vi "Test LakeShore 340.vi"(8 "error in (no error)":errorcluster, 11 "VISA Resource Name":refnum<visa-resource-name>) -> (0 "error out":errorcluster, 2 "Heater%":dbl, 3 "VISA Resource Name Out":refnum<visa-resource-name>)   [LabVIEW 2024]
panel:
  out "read buffer":string
  in  "byte count":u32
  out "Raw 2":dbl
  out "Temperature 2":dbl
  in  "Set point":dbl format="%.2f"
  in  "Output #":i32=1
  out "Raw":dbl
  out "Temperature":dbl
  in  "Input (A or B)":string="A"
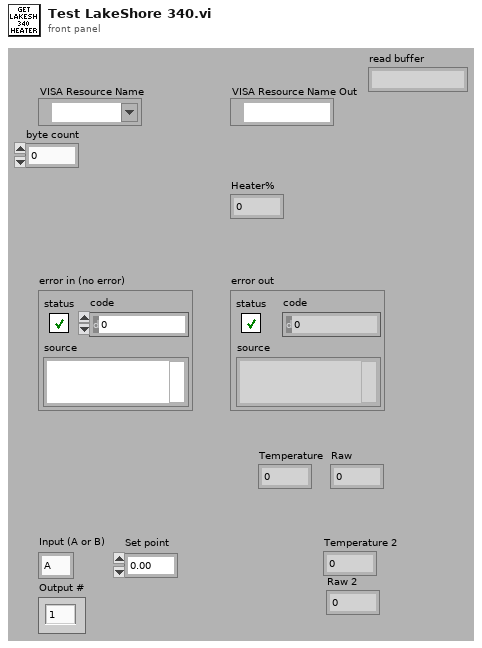
[diagram p1: front panel]
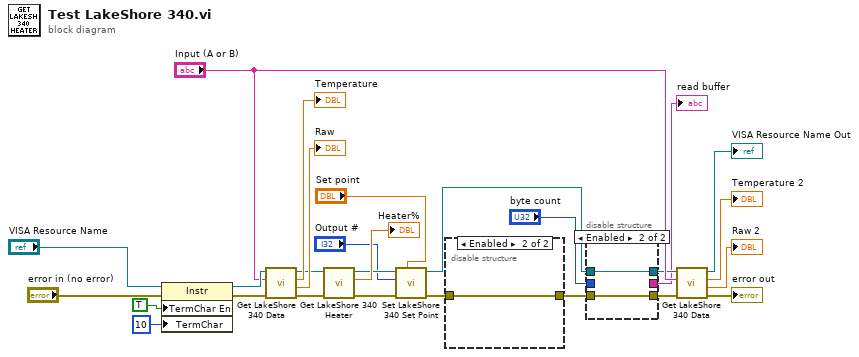
[diagram p0: block diagram]
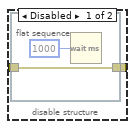
[diagram p2: hidden frame]
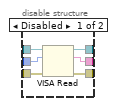
[diagram p3: hidden frame]
diagram:
  n1 = property class="Instr"(reference="VISA Resource Name", error in="error in (no error)", "TermChar En"=TRUE ("Message Based Settings:Termination Character Enable"), "TermChar"=u8 10 ("Message Based Settings:Termination Character")) -> (reference out=w23:refnum<visa-resource-name>, error out=w22:errorcluster)
  n2 = call "Get LakeShore 340 Data.vi"("error in (no error)"=w22, "Input (A or B)"="Input (A or B)", "VISA Resource Name"=w23) -> ("error out"=w18:errorcluster, "Raw"=→"Raw":dbl, "Temperature"=→"Temperature":dbl, "VISA Resource Name Out"=w19:refnum<visa-resource-name>)  [unwired: 5 in]
  n3 = call "Get LakeShore 340 Heater.vi"("error in (no error)"=w18, "VISA Resource Name"=w19) -> ("error out"=w16:errorcluster, "Heater%"=→"Heater%":dbl, "VISA Resource Name Out"=w14:refnum<visa-resource-name>)  [unwired: 7 in]
  n4 = call "Set LakeShore 340 Set Point.vi"("Set point"="Set point", "error in (no error)"=w16, "Output #"="Output #", "VISA Resource Name"=w14) -> ("error out"=w7:errorcluster, "VISA Resource Name Out"=w6:refnum<visa-resource-name>)  [unwired: 6 in]
  n5 = disable-structure shown="Enabled" {
    disable-tunnel: w7 -> [w29 w32]
    disable-tunnel: [w28 w32] -> w5
    frame Disabled {
      n6 = flat-sequence {
        tunnel: [w30] -> w28
        tunnel: w29 -> [w30]
        frame #0 {
          n7 = Wait (ms)(milliseconds to wait=u32 1000) -> ()  [unwired: 1 out]
        }
      }
    }
    frame Enabled {
    }
  }
  n8 = disable-structure shown="Enabled" {
    disable-tunnel: w6 -> [w38 w40]
    disable-tunnel: w5 -> [w37 w39]
    disable-tunnel: [w36 w40] -> w4
    disable-tunnel: [w35 w39] -> w3
    disable-tunnel: "byte count" -> [w34 _]
    disable-tunnel: [w33 _] -> w1
    frame Disabled {
      n9 = VISA Read(VISA resource name=w38, byte count=w34, error in (no error)=w37) -> (VISA resource name out=w36:refnum<visa-resource-name>, read buffer=w33:string, error out=w35:errorcluster)  [unwired: 1 out]
    }
    frame Enabled {
    }
  }
  "read buffer" <- w1
  n10 = call "Get LakeShore 340 Data.vi"("error in (no error)"=w3, "Input (A or B)"="Input (A or B)", "VISA Resource Name"=w4) -> ("error out"=→"error out":errorcluster, "Raw"=→"Raw 2":dbl, "Temperature"=→"Temperature 2":dbl, "VISA Resource Name Out"=→"VISA Resource Name Out":refnum<visa-resource-name>)  [unwired: 5 in]
